vi "XMLGetAttributeVal.vi"(8 "error in":errorcluster, 10 "Attribute XPath":string, 11 "Node In":refnum<k20>) -> (0 "error out":errorcluster, 2 "Value":string, 3 "Node out":refnum<k20>)   [LabVIEW 2011]
uses:
  <vilib>/xml/NI_XML.lvlib
  Program Files (x86)/National Instruments/LabVIEW 2011/resource/objmgr/DOMUserDefRef.rc
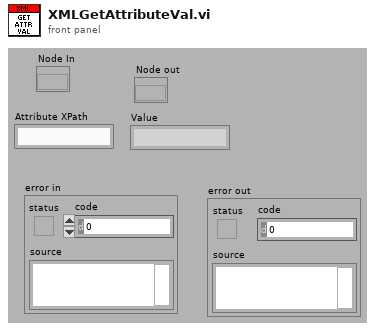
[diagram p1: front panel]
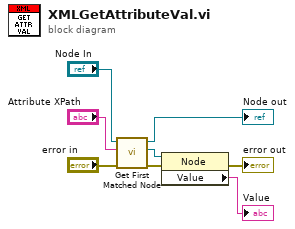
[diagram p0: block diagram]
diagram:
  n1 = call <vilib>:"Get First Matched Node.vi"("error in (no error)"="error in", "XPath expression"="Attribute XPath", "node in"="Node In") -> ("error out"=w4:errorcluster, "node result"=w6:refnum<k20>, "node out"=→"Node out":refnum<k20>)  [unwired: 6 in]
  n2 = property class="Node"(reference=w6, error in=w4) -> (error out=→"error out":errorcluster, "Value"=→"Value":string)  [unwired: 1 out]
